vi "Lab 2 Q1.vi"() -> ()   [LabVIEW 2016]
panel:
  out "Waveform Chart":dbl(graph)
  out "Sum":dbl
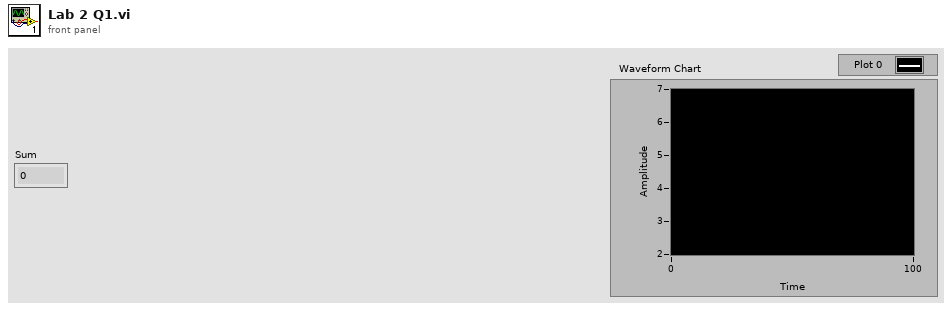
[diagram p1: front panel]
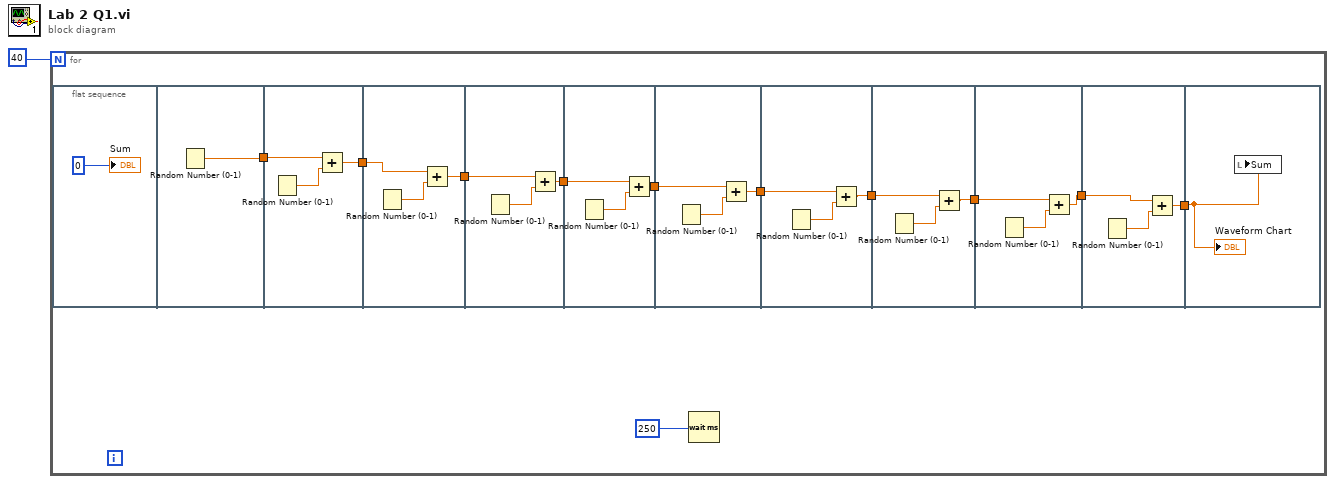
[diagram p0: block diagram]
diagram:
  n1 = for {
    N: 40 -> [_]
    n2 = flat-sequence {
      tunnel: [w14] -> w11
      tunnel: w11 -> [w17]
      tunnel: [w15] -> w9
      tunnel: [w19] -> w10
      tunnel: w9 -> [w18]
      tunnel: w10 -> [w22]
      tunnel: [w21] -> w8
      tunnel: w8 -> [w25]
      tunnel: [w24] -> w7
      tunnel: w7 -> [w28]
      tunnel: [w27] -> w6
      tunnel: w6 -> [w31]
      tunnel: [w30] -> w5
      tunnel: w5 -> [w34]
      tunnel: [w33] -> w4
      tunnel: w4 -> [w37]
      tunnel: [w36] -> w3
      tunnel: w3 -> [w40]
      tunnel: [w39] -> w2
      tunnel: w2 -> [w42]
      frame #0 {
        "Sum" <- 0
      }
      frame #1 {
        n3 = Random Number (0-1)() -> (number: 0 to 1=w14:dbl)
      }
      frame #2 {
        n4 = Random Number (0-1)() -> (number: 0 to 1=w16:dbl)
        n5 = Add(x=w17, y=w16) -> (x+y=w15:dbl)
      }
      frame #3 {
        n6 = Random Number (0-1)() -> (number: 0 to 1=w20:dbl)
        n7 = Add(x=w18, y=w20) -> (x+y=w19:dbl)
      }
      frame #4 {
        n8 = Random Number (0-1)() -> (number: 0 to 1=w23:dbl)
        n9 = Add(x=w22, y=w23) -> (x+y=w21:dbl)
      }
      frame #5 {
        n10 = Random Number (0-1)() -> (number: 0 to 1=w26:dbl)
        n11 = Add(x=w25, y=w26) -> (x+y=w24:dbl)
      }
      frame #6 {
        n12 = Random Number (0-1)() -> (number: 0 to 1=w29:dbl)
        n13 = Add(x=w28, y=w29) -> (x+y=w27:dbl)
      }
      frame #7 {
        n14 = Random Number (0-1)() -> (number: 0 to 1=w32:dbl)
        n15 = Add(x=w31, y=w32) -> (x+y=w30:dbl)
      }
      frame #8 {
        n16 = Random Number (0-1)() -> (number: 0 to 1=w35:dbl)
        n17 = Add(x=w34, y=w35) -> (x+y=w33:dbl)
      }
      frame #9 {
        n18 = Random Number (0-1)() -> (number: 0 to 1=w38:dbl)
        n19 = Add(x=w37, y=w38) -> (x+y=w36:dbl)
      }
      frame #10 {
        n20 = Random Number (0-1)() -> (number: 0 to 1=w41:dbl)
        n21 = Add(x=w40, y=w41) -> (x+y=w39:dbl)
      }
      frame #11 {
        n22 = local write "Sum"(w42) -> ()
        "Waveform Chart" <- w42
      }
    }
    n23 = Wait (ms)(milliseconds to wait=250) -> ()  [unwired: 1 out]
  }
